vi "Set Name at Path.vi"(0 "Variant in":variant, 5 "Path String":string, 9 "Name":string, 11 "error in (no error)":errorcluster) -> (4 "Variant out":variant, 15 "error out":errorcluster)   [LabVIEW 2017, in "Advanced Variant Tools.lvlib"]
uses:
  Advanced Variant Tools.lvlib
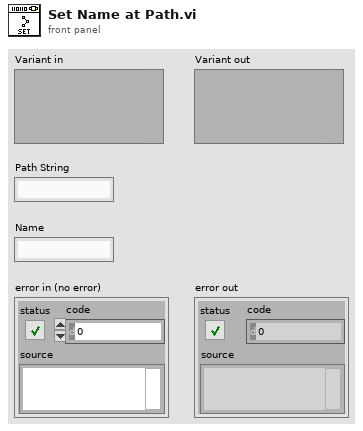
[diagram p1: front panel]
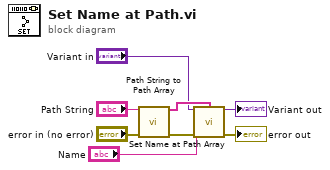
[diagram p0: block diagram]
diagram:
  n1 = call "Path String to Path Array.vi"("Path String"="Path String", "error in (no error)"="error in (no error)") -> ("array"=w7:string[], "error out"=w8:errorcluster)  [unwired: 12 in]
  n2 = call "Set Name at Path Array.vi"("Variant in"="Variant in", "Path in"=w7, "Name"="Name", "error in (no error)"=w8) -> ("Variant out"=→"Variant out":variant, "error out"=→"error out":errorcluster)  [unwired: 10 in]
